vi "FTW-Actor-QueryConfigurationParameter.vi"(0 "FTW Actor":refnum<class "FTW-Actor.lvclass">, 5 "Config Parameter (Type and Default)":string, 11 "error in":errorcluster) -> (4 "FTW Actor out":refnum<class "FTW-Actor.lvclass">, 6 "Value":string, 15 "error out":errorcluster)   [LabVIEW 2014, in "FTW-Actor.lvclass"]
uses:
  FTW-Actor.lvclass
  Container/FTW-Container.lvclass
panel:
  # "Inputs"
  # "Outputs"
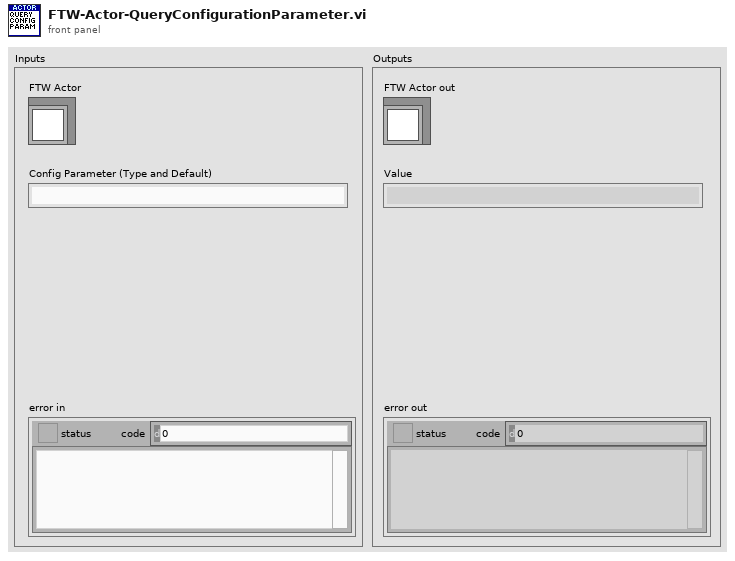
[diagram p1: front panel]
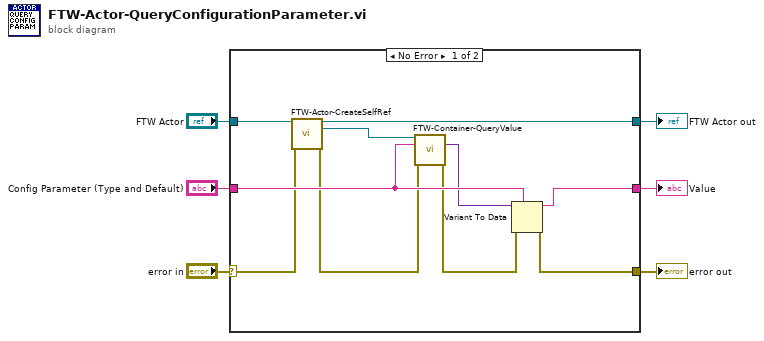
[diagram p0: block diagram]
diagram:
  n1 = case shown="No Error" "error in" {
    selector: "error in" -> [w8 w17]
    tunnel: [w16 w17] -> w6
    tunnel: "FTW Actor" -> [w11 w19]
    tunnel: [w10 w19] -> w4
    tunnel: "Config Parameter (Type and Default)" -> [w15 w18]
    tunnel: [w14 w18] -> w2
    frame No Error {
      n2 = call "FTW-Actor-CreateSelfRef.vi"("FTW Actor"=w11, "error in"=w8) -> ("FTW Actor out"=w10:refnum<class "FTW-Actor.lvclass">, "Reference to Self"=w9:refnum<class "FTW-ActorReference.lvclass">, "error out"=w7:errorcluster)  [unwired: 11 in]
      n3 = call "FTW-Container-QueryValue.vi"("Container"=w9, "Type and Defaults"=w15, "error in"=w7) -> ("Result"=w12:variant, "error out"=w13:errorcluster)  [unwired: 10 in, 1 out]
      n4 = Variant To Data(error in=w13, type=w15, Variant=w12) -> (data=w14:string, error out=w16:errorcluster)
    }
    frame Error {
    }
  }
  "error out" <- w6
  "FTW Actor out" <- w4
  "Value" <- w2
